vi "数据回放 - v1.1.vi"() -> ()   [LabVIEW 2020]
panel:
  out "发动机运行参数 2":waveform(dbl)[](graph)=[{"t0"=timestamp(3721454179.1141996 s since 1904-01-01), "dt"=0.1, "Y"=[0.0], "attributes"=variant("NI_ChannelName"=variant(string "滤波"), "NI_ExpIsRelativeTime"=variant(bool FALSE), "NI_ExpStartTimeStamp"=variant(timestamp timestamp(3721452975.9819994 s since 1904-01-01)), "NI_ExpTimeStamp"=variant(timestamp timestamp(3721452977.9214687 s since 1904-01-01)), "NI_ExpXDimension"=variant(string "t"), "NI_UnitDescription"=variant(string "V"))}, {"t0"=timestamp(3721454179.1141996 s since 1904-01-01), "dt"=0.1, "Y"=[0.0], "attributes"=variant("NI_ChannelName"=variant(string "滤波 1"), "NI_ExpIsRelativeTime"=variant(bool FALSE), "NI_ExpStartTimeStamp"=variant(timestamp timestamp(3721452975.9819994 s since 1904-01-01)), "NI_ExpTimeStamp"=variant(timestamp timestamp(3721452977.9214687 s since 1904-01-01)), "NI_ExpXDimension"=variant(string "t"), "NI_UnitDescription"=variant(string "V"))}, {"t0"=timestamp(3721454179.1141996 s since 1904-01-01), "dt"=0.1, "Y"=[195137.511642], "attributes"=variant("NI_ChannelName"=variant(string "滤波 2"), "NI_ExpIsRelativeTime"=variant(bool FALSE), "NI_ExpStartTimeStamp"=variant(timestamp timestamp(3721452975.9819994 s since 1904-01-01)), "NI_ExpTimeStamp"=variant(timestamp timestamp(3721452977.9214687 s since 1904-01-01)), "NI_ExpXDimension"=variant(string "t"), "NI_UnitDescription"=variant(string "V"))}, {"t0"=timestamp(3721454179.1141996 s since 1904-01-01), "dt"=0.1, "Y"=[15.560715], "attributes"=variant("NI_ChannelName"=variant(string "滤波 3"), "NI_ExpIsRelativeTime"=variant(bool FALSE), "NI_ExpStartTimeStamp"=variant(timestamp timestamp(3721452975.9819994 s since 1904-01-01)), "NI_ExpTimeStamp"=variant(timestamp timestamp(3721452977.9214687 s since 1904-01-01)), "NI_ExpXDimension"=variant(string "t"), "NI_UnitDescription"=variant(string "V"))}, {"t0"=timestamp(3721454179.1141996 s since 1904-01-01), "dt"=0.1, "Y"=[15.568908], "attributes"=variant("NI_ChannelName"=variant(string "滤波 4"), "NI_ExpIsRelativeTime"=variant(bool FALSE), "NI_ExpStartTimeStamp"=variant(timestamp timestamp(3721452975.9819994 s since 1904-01-01)), "NI_ExpTimeStamp"=variant(timestamp timestamp(3721452977.9214687 s since 1904-01-01)), "NI_ExpXDimension"=variant(string "t"), "NI_UnitDescription"=variant(string "V"))}]
  in  "Filename":path=path "test.lvm" caption="发动机参数"
  # "数据回放V1.1"
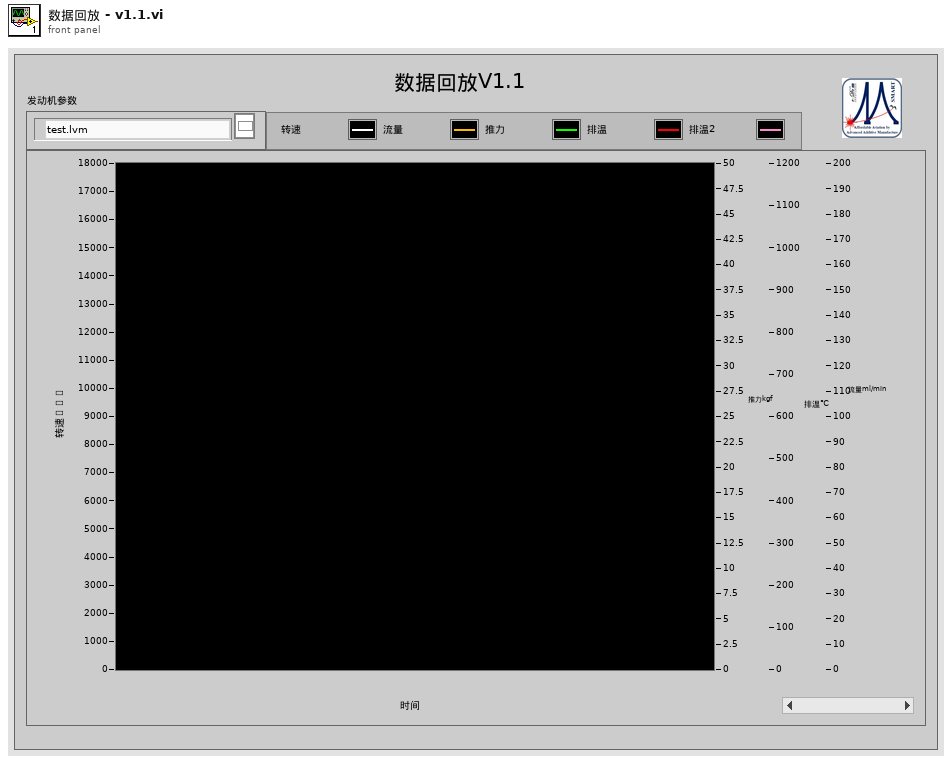
[diagram p1: front panel]
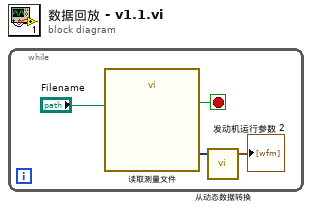
[diagram p0: block diagram]
diagram:
  n1 = while {
    stop <- w3 stop-if-true
    n2 = call "读取测量文件"("Filename"="Filename") -> ("Signals"=w2:dynamicdata, "EOF?"=w3:bool)  [unwired: 5 in, 4 out]
    n3 = call "从动态数据转换"("Dynamic Data Type"=w2) -> ("Array of Waveform"=→"发动机运行参数 2":waveform(dbl)[])  [unwired: 3 in]
  }
